vi "Define macro contents.vi"(0 "System no.":i32=1 min=1 max=4 step=1, 2 "Macro contents":string, 5 "error in":errorcluster) -> (19 "error out":errorcluster)   [LabVIEW 2026]
doc: "Defines macro contents. Each command to be stored in the macro must be written on one line, terminated with the enter key. MAC BEG.vi must be called before running this VI and MAC END.vi must be called afterwards.\n\nE-816: Macro will not be saved to FLASH until WPA .vi was run. Changes not saved with WPA are only present in RAM and will be lost when the controller is powered off. This command cannot be issued to a slave. Check controller manual to find out if MAC is supported.\n\nM-8X0: Only for GCS syntax version = GCS 2.0 or higher (check with CSV?.vi. If CSV?.vi is not supported, syntax version is GCS 1.0)."
panel:
  out "Array":string[](array[string])
  # "Defines macro contents. Each command to be stored in the macro must\nbe written on one line, terminated with the enter key. MAC BEG.vi must \nbe called before running this VI and MAC END.vi must be called afterwards.\nVI sends Macro contents one line after another separated by the specified\nwait time."
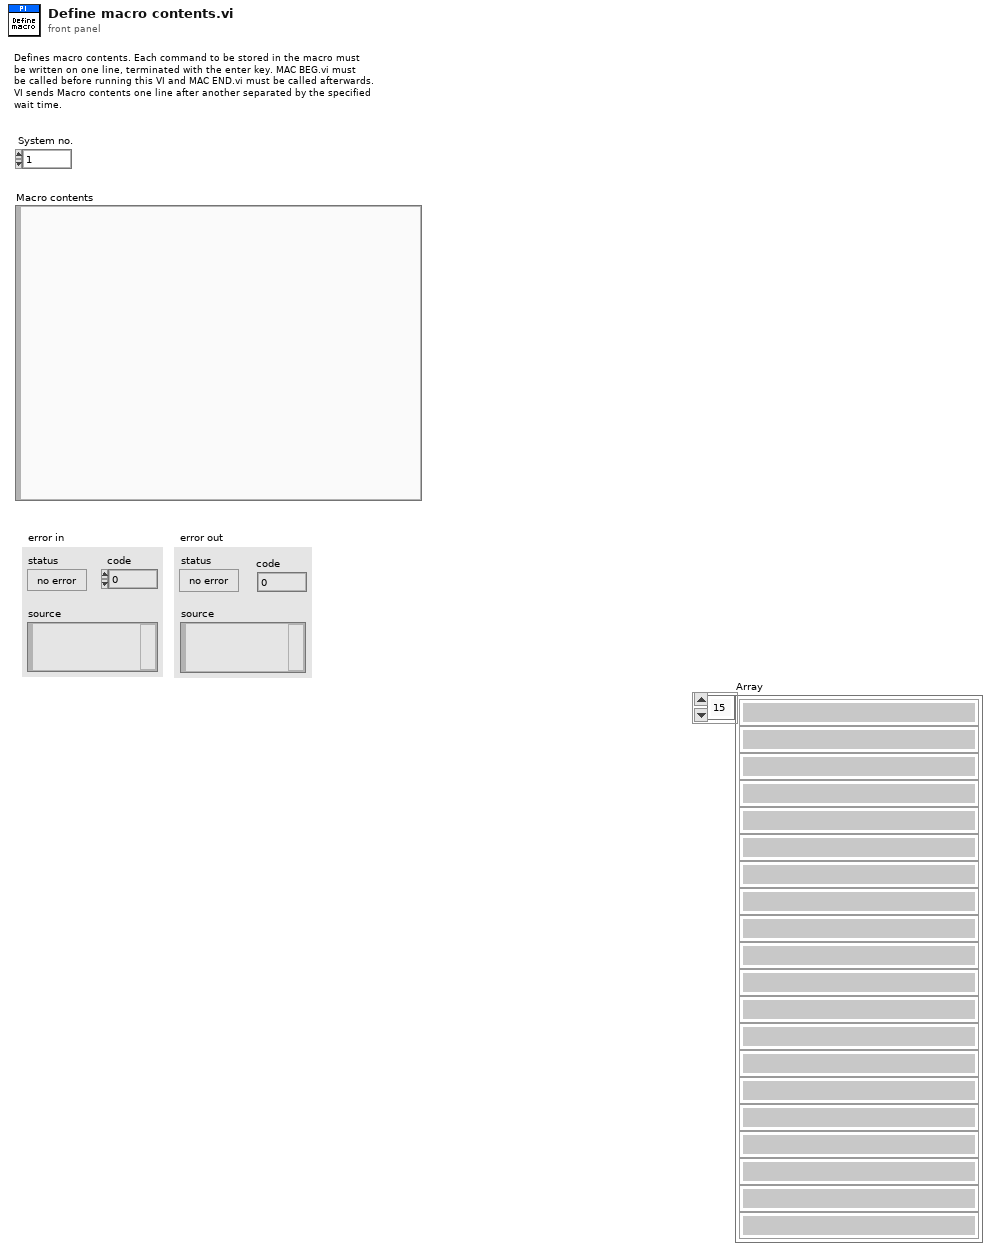
[diagram p1: front panel]
types:
  T1 = enum16{"Disable error check", "Force error check", "Use global settings"}
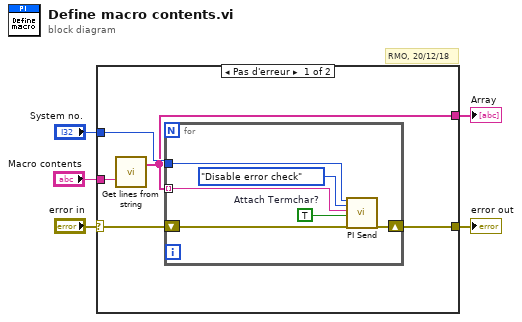
[diagram p0: block diagram]
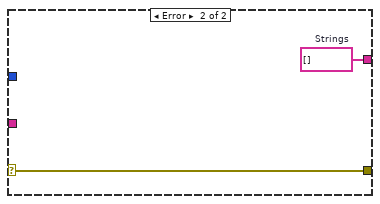
[diagram p2: hidden frame]
diagram:
  # "RMO, 20/12/18"
  n1 = case shown="Pas d'erreur" "error in" {
    selector: "error in" -> [w6 w18]
    tunnel: "System no." -> [w10 _]
    tunnel: [w9 w18] -> w4
    tunnel: "Macro contents" -> [w8 _]
    tunnel: [w7 w17] -> w2
    frame No Error {
      n2 = call "Get lines from string.vi"("Input string"=w8) -> ("Strings"=w7:string[])  [unwired: 2 in, 16 out]
      n3 = for {
        tunnel: w7 -> [w14] mode=indexing
        tunnel: w10 -> [w13]
        shift-right: [w16] -> w9
        shift-left: w6 -> [w12]
        w15 = TRUE  # Attach Termchar?
        n4 = call "PI Send.vi"("System no."=w13, "Error check settings"=T1."Disable error check", "String to send"=w14, "Attach termination char.?"=w15, "error in"=w12) -> ("error out"=w16:errorcluster)  [unwired: 1 in, 13 out]
      }
    }
    frame Error {
      w17 = string[] []  # Strings
    }
  }
  "Array" <- w2
  "error out" <- w4
